vi "sub_DTMF_BitPadding.vi"(9 "Modulation Order":i8=4, 11 "TXbitStream":i8[](array[numeric])) -> (3 "TXbitStream Output":i8[](array[numeric]), 5 "PaddingBits":i8)   [LabVIEW 2011]
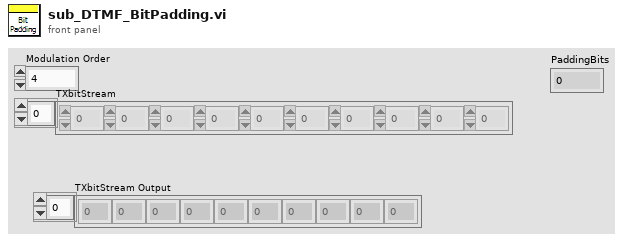
[diagram p1: front panel]
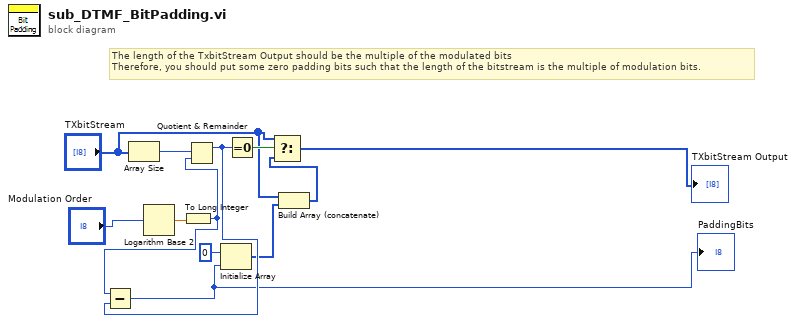
[diagram p0: block diagram]
diagram:
  # "The length of the TxbitStream Output should be the multiple of the modulated bits\nTherefore, you should put some zero padding bits such that the length of the bitstream is the multiple of modulation bits."
  n1 = Array Size(array="TXbitStream") -> (size(s)=w12:i32)
  n2 = Logarithm Base 2(1:"Modulation Order") -> (0:w10:dbl)
  n3 = To Long Integer(number=w10) -> (32bit integer=w5:i32)
  n4 = Quotient & Remainder(x=w12, y=w5) -> (x-y*floor(x/y)=w4:i32)  [unwired: 1 out]
  n5 = Subtract(x=w5, y=w4) -> (x-y=w1:i32)
  "PaddingBits" <- w1
  n6 = Initialize Array(0 ("element"), w1) -> (w3:i32[])
  n7 = Equal To 0?(x=w4) -> (x = 0?=w9:bool)
  n8 = Build Array (concatenate)("TXbitStream", w3) -> (w2:i32[])
  n9 = Select(t="TXbitStream", s=w9, f=w2) -> (s? t:f=→"TXbitStream Output":i32[])
